vi "FPGA Main.vi"() -> ()   [LabVIEW 2009]
uses:
  FPGA Opperation Mode.ctl
  Motor Control/Motor Output Global.vi
  Motor Control/Motor Encoder Global.vi
  Motor Control/Inner Control/Drive Control Global DO NOT MODIFY!.vi
panel:
  in  "Enum":T1
  in  "Steering Position Offset":i32
  out "Drive Encoder ft/sec":fxp<+/-,18,8>
  in  "Drive Enable":bool
  in  "Drive Speed Current (1-3.5)":fxp<+/-,18,8>
  in  "Stop":bool
  in  "Steering Proportional Control Feedback Gain":fxp<+/-,20,5>
  in  "Steering Enable":bool
  in  "Steering Position Target":i32
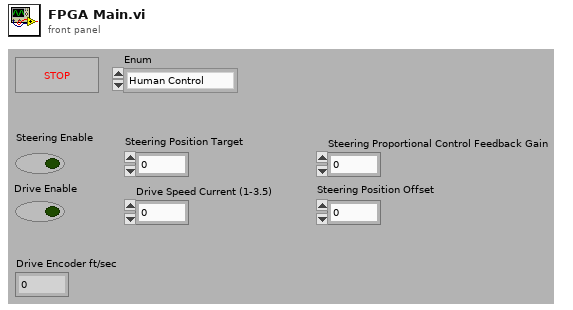
[diagram p1: front panel]
types:
  T1 = typedef "FPGA Opperation Mode.ctl" = enum16{"Human Control"}
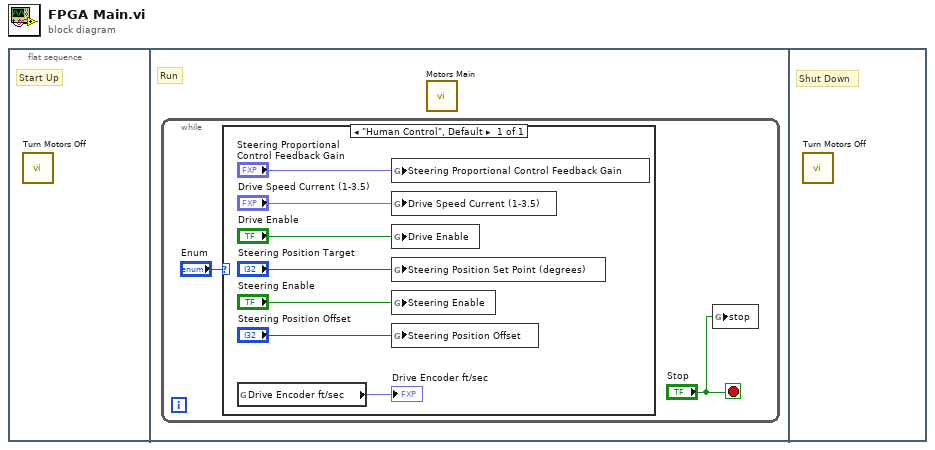
[diagram p0: block diagram]
diagram:
  n1 = flat-sequence {
    frame #0 {
      # "Start Up"
      n2 = call "Turn Motors Off.vi"() -> ()  [unwired: 1 in]
    }
    frame #1 {
      # "Run"
      n3 = while {
        stop <- "Stop" stop-if-true
        n4 = case shown="\"Human Control\", Default" "Enum" {
          frame "Human Control", Default {
            n5 = global read "Drive Control Global DO NOT MODIFY!.vi" "Drive Encoder ft/sec"() -> (→"Drive Encoder ft/sec":fxp<+/-,18,8>)
            n6 = global write "Motor Encoder Global.vi" "Steering Proportional Control Feedback Gain"("Steering Proportional Control Feedback Gain") -> ()
            n7 = global write "Motor Encoder Global.vi" "Drive Speed Current (1-3.5)"("Drive Speed Current (1-3.5)") -> ()
            n8 = global write "Motor Output Global.vi" "Drive Enable"("Drive Enable") -> ()
            n9 = global write "Motor Encoder Global.vi" "Steering Position Set Point (degrees)"("Steering Position Target") -> ()
            n10 = global write "Motor Output Global.vi" "Steering Enable"("Steering Enable") -> ()
            n11 = global write "Motor Encoder Global.vi" "Steering Position Offset"("Steering Position Offset") -> ()
          }
        }
        n12 = global write "Motor Encoder Global.vi" "stop"("Stop") -> ()
      }
      n13 = call "Motors Main.vi"() -> ()  [unwired: 1 in]
    }
    frame #2 {
      # "Shut Down"
      n14 = call "Turn Motors Off.vi"() -> ()  [unwired: 1 in]
    }
  }
